vi "Configure Module.vi"(8 "error in":errorcluster, 10 "IOV ref in":refnum<k21>, 11 "9253 in":refnum<class "9253.lvclass">) -> (0 "error out":errorcluster, 2 "IOV ref out":refnum<k21>, 3 "9253 out":refnum<class "9253.lvclass">)   [LabVIEW 2017, in "Modules.lvlib" / "9253.lvclass"]
uses:
  9253.lvclass
  C:/Users/nitest/Documents/NI/niveristand-scan-engine-module-libraries/Source/RSI Module/RSI Module.lvclass
  9253.lvclass/9253.ctl
  <resource>/objmgr/cRIO.rc
  RSI Module/RSI Module.lvclass
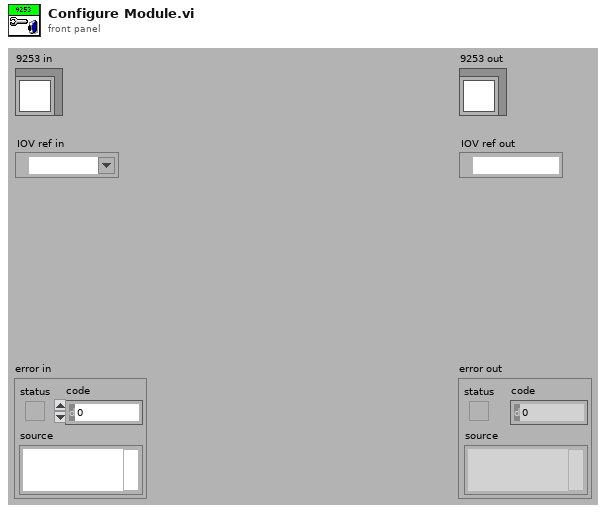
[diagram p1: front panel]
types:
  T1 = cluster{"fault detection enable":bool, "lower fault detection limit":dbl, "upper fault detection limit":dbl}[]
  T2 = typedef "Modules.lvlib/RSI Module.lvclass/Channels.ctl" = cluster{"# Input Channels":i32, "# Output Channels":i32, "Channel Type":T3, "Units":string}
  T3 = typedef "Modules.lvlib/RSI Module.lvclass/Channel Type.ctl" = enum16{"Analog", "Digital"}
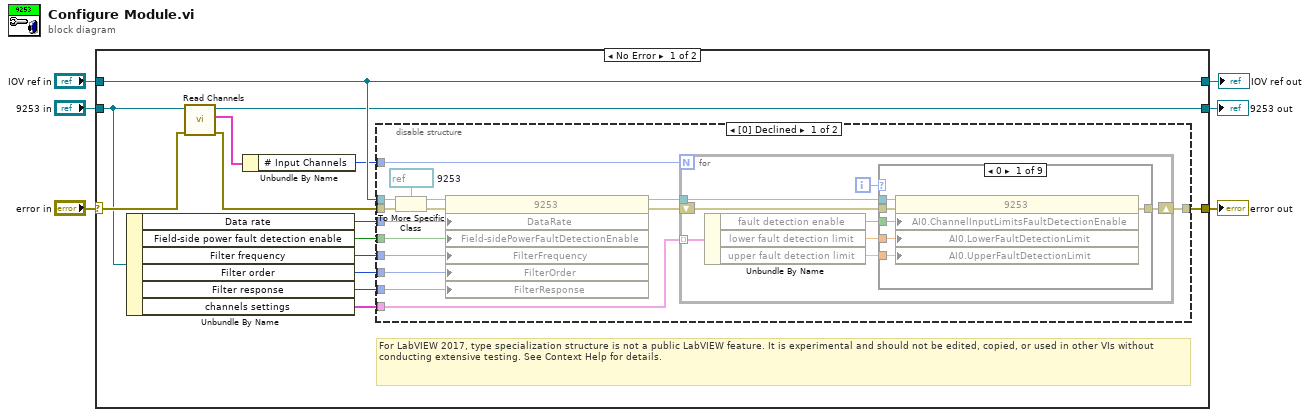
[diagram p0: block diagram]
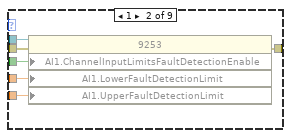
[diagram p2: hidden frame]
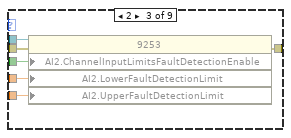
[diagram p3: hidden frame]
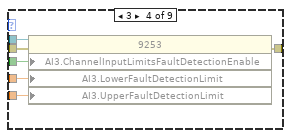
[diagram p4: hidden frame]
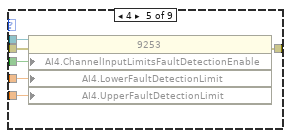
[diagram p5: hidden frame]
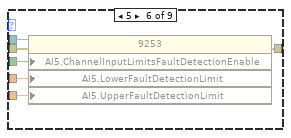
[diagram p6: hidden frame]
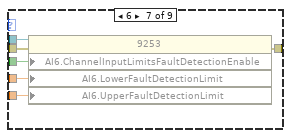
[diagram p7: hidden frame]
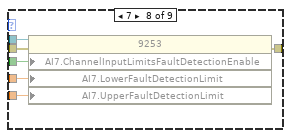
[diagram p8: hidden frame]
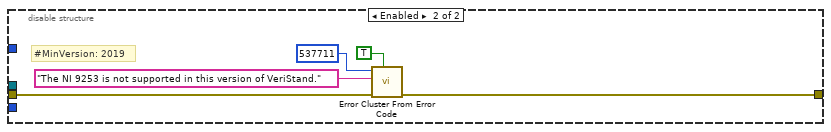
[diagram p10: hidden frame]
diagram:
  n1 = case shown="No Error" "error in" {
    selector: "error in" -> [w11 w100]
    tunnel: [w19 w100] -> w5
    tunnel: [w12 w99] -> w3
    tunnel: "9253 in" -> [w7 w99]
    tunnel: "IOV ref in" -> [w20 w98]
    tunnel: [w20 w98] -> w1
    frame No Error {
      # "For LabVIEW 2017, type specialization structure is not a public LabVIEW feature. It is experimental and should not be edited, copied, or used in other VIs without conducting extensive testing. See Context Help for details."
      n2 = Unbundle By Name(w7) -> ("Data rate"=w18:u32, "Field-side power fault detection enable"=w17:bool, "Filter frequency"=w16:u32, "Filter order"=w15:u32, "Filter response"=w14:u32, "channels settings"=w13:T1)
      n3 = call "Read Channels.vi"("error in (no error)"=w11, "RSI Module in"=w7) -> ("error out"=w10:errorcluster, "Channels"=w9:T2, "RSI Module out"=w12:refnum<class "9253.lvclass">)  [unwired: 7 in]
      n4 = Unbundle By Name(w9) -> ("# Input Channels"=w8:i32)
      n5 = disable-structure shown="[0] Declined" {
        disable-tunnel: w10 -> [w30 w94]
        disable-tunnel: [w29 w93] -> w19
        disable-tunnel: w20 -> [w28 _]
        disable-tunnel: w18 -> [w27 _]
        disable-tunnel: w17 -> [w26 _]
        disable-tunnel: w16 -> [w25 _]
        disable-tunnel: w15 -> [w24 _]
        disable-tunnel: w14 -> [w23 _]
        disable-tunnel: w13 -> [w22 _]
        disable-tunnel: w8 -> [w21 _]
        frame Disabled {
          w35 = refnum<k21> refnum  # 9253
          n6 = To More Specific Class(target class=w35, reference=w28, error in=w30) -> (specific class reference=w34:refnum<k21>, error out=w33:errorcluster)
          n7 = property class="9253"(reference=w34, error in=w33, "DataRate"=w27, "Field-sidePowerFaultDetectionEnable"=w26, "FilterFrequency"=w25, "FilterOrder"=w24, "FilterResponse"=w23) -> (reference out=w32:refnum<k21>, error out=w31:errorcluster)
          n8 = for {
            N: w21 -> [_]
            tunnel: w32 -> [w42]
            shift-right: [w43] -> w29
            shift-left: w31 -> [w41]
            tunnel: w22 -> [w39] mode=indexing
            i -> [w40]
            n9 = Unbundle By Name(w39) -> ("fault detection enable"=w38:bool, "lower fault detection limit"=w37:dbl, "upper fault detection limit"=w36:dbl)
            n10 = case shown="0" w40 {
              tunnel: [w49 w55 w61 w67 w73 w79 w85 w91 w92] -> w43
              tunnel: w38 -> [w48 w54 w60 w66 w72 w78 w84 w90 _]
              tunnel: w37 -> [w47 w53 w57 w63 w69 w75 w81 w87 _]
              tunnel: w36 -> [w46 w52 w56 w62 w68 w74 w80 w86 _]
              tunnel: w42 -> [w45 w51 w59 w65 w71 w77 w83 w89 _]
              tunnel: w41 -> [w44 w50 w58 w64 w70 w76 w82 w88 w92]
              frame 0 {
                n11 = property class="9253"(reference=w45, error in=w44, "AI0.ChannelInputLimitsFaultDetectionEnable"=w48, "AI0.LowerFaultDetectionLimit"=w47, "AI0.UpperFaultDetectionLimit"=w46) -> (error out=w49:errorcluster)  [unwired: 1 out]
              }
              frame 1 {
                n12 = property class="9253"(reference=w51, error in=w50, "AI1.ChannelInputLimitsFaultDetectionEnable"=w54, "AI1.LowerFaultDetectionLimit"=w53, "AI1.UpperFaultDetectionLimit"=w52) -> (error out=w55:errorcluster)  [unwired: 1 out]
              }
              frame 2 {
                n13 = property class="9253"(reference=w59, error in=w58, "AI2.ChannelInputLimitsFaultDetectionEnable"=w60, "AI2.LowerFaultDetectionLimit"=w57, "AI2.UpperFaultDetectionLimit"=w56) -> (error out=w61:errorcluster)  [unwired: 1 out]
              }
              frame 3 {
                n14 = property class="9253"(reference=w65, error in=w64, "AI3.ChannelInputLimitsFaultDetectionEnable"=w66, "AI3.LowerFaultDetectionLimit"=w63, "AI3.UpperFaultDetectionLimit"=w62) -> (error out=w67:errorcluster)  [unwired: 1 out]
              }
              frame 4 {
                n15 = property class="9253"(reference=w71, error in=w70, "AI4.ChannelInputLimitsFaultDetectionEnable"=w72, "AI4.LowerFaultDetectionLimit"=w69, "AI4.UpperFaultDetectionLimit"=w68) -> (error out=w73:errorcluster)  [unwired: 1 out]
              }
              frame 5 {
                n16 = property class="9253"(reference=w77, error in=w76, "AI5.ChannelInputLimitsFaultDetectionEnable"=w78, "AI5.LowerFaultDetectionLimit"=w75, "AI5.UpperFaultDetectionLimit"=w74) -> (error out=w79:errorcluster)  [unwired: 1 out]
              }
              frame 6 {
                n17 = property class="9253"(reference=w83, error in=w82, "AI6.ChannelInputLimitsFaultDetectionEnable"=w84, "AI6.LowerFaultDetectionLimit"=w81, "AI6.UpperFaultDetectionLimit"=w80) -> (error out=w85:errorcluster)  [unwired: 1 out]
              }
              frame 7 {
                n18 = property class="9253"(reference=w89, error in=w88, "AI7.ChannelInputLimitsFaultDetectionEnable"=w90, "AI7.LowerFaultDetectionLimit"=w87, "AI7.UpperFaultDetectionLimit"=w86) -> (error out=w91:errorcluster)  [unwired: 1 out]
              }
              frame Default {
              }
            }
          }
        }
        frame Enabled {
          # "#MinVersion: 2019"
          n19 = call <vilib>:"Error Cluster From Error Code.vi"("show call chain? (False)"=TRUE, "error in (no error)"=w94, "error message (\"\")"="The NI 9253 is not supported in this version of VeriStand." ("error message (\"\")"), "error code (0)"=537711) -> ("error out"=w93:errorcluster)  [unwired: 5 in]
        }
      }
    }
    frame Error {
    }
  }
  "error out" <- w5
  "9253 out" <- w3
  "IOV ref out" <- w1
